vi "Scaling Test.vi"() -> ()   [LabVIEW 2016]
panel:
  out "Pre-Twos":bool[](array[boolean])
  out "Two's Complement":bool[](array[boolean])
  in  "Bit Count":u8=12
  out "Raw U64":u64 format="%064b"
  in  "Direction":bool
  in  "Raw":u16[](array[numeric]) format="%016b"
  in  "Scaled":dbl
  in  "Bit Offset":u8=2
  in  "LSB Resolution":dbl=1.0
  in  "2's Complement":bool
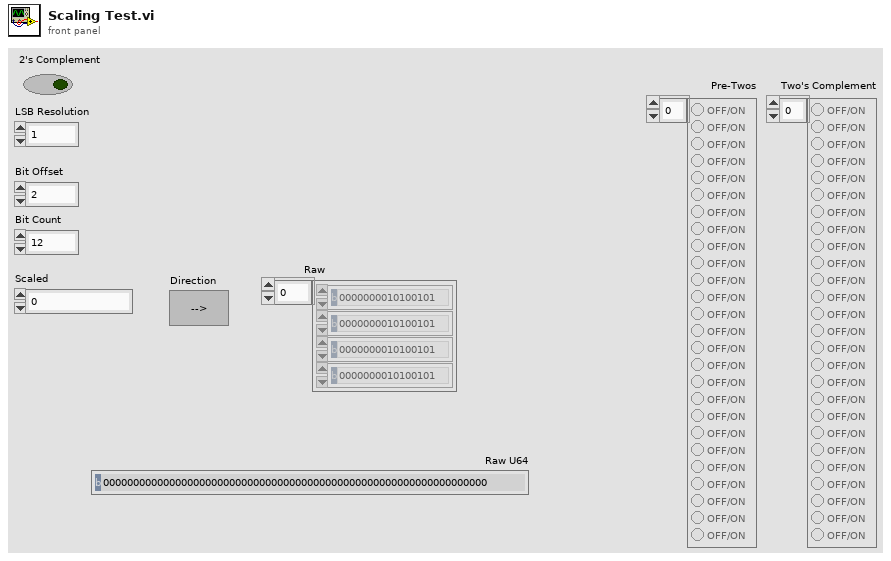
[diagram p1: front panel]
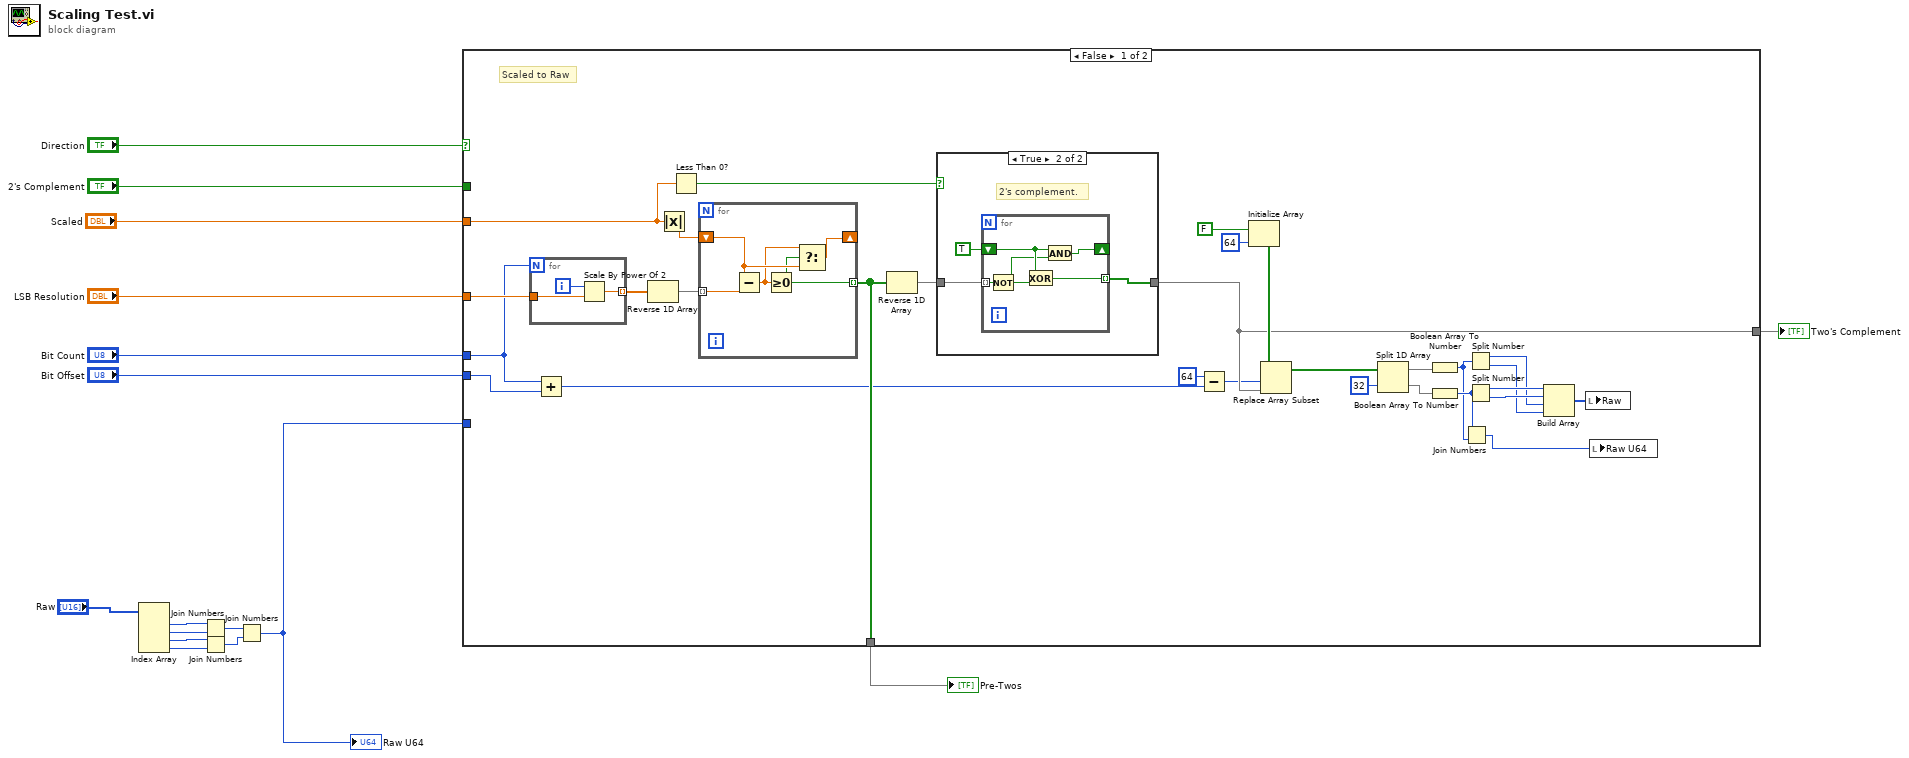
[diagram p0: block diagram]
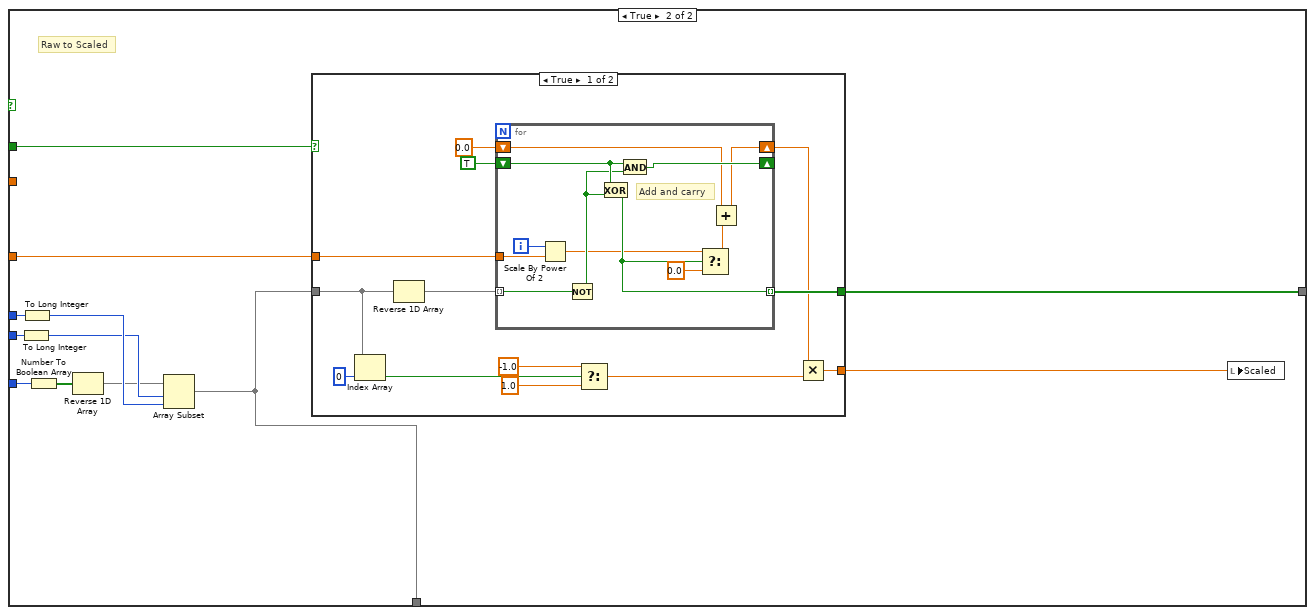
[diagram p3: hidden frame]
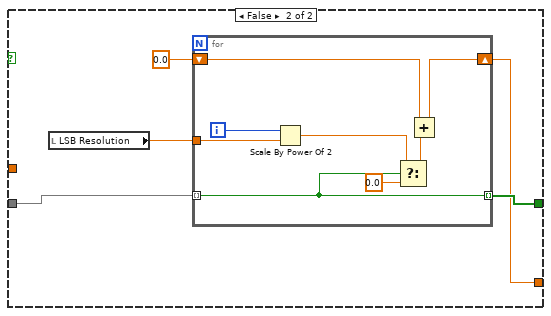
[diagram p4: hidden frame]
diagram:
  n1 = Index Array(array="Raw") -> (element #1=w6:u16, element #2=w7:u16, element #3=w4:u16, element #4=w5:u16)  [unwired: 4 in]
  n2 = Join Numbers(hi=w6, lo=w7) -> ((hi.lo)=w2:u32)
  n3 = Join Numbers(hi=w4, lo=w5) -> ((hi.lo)=w3:u32)
  n4 = Join Numbers(hi=w2, lo=w3) -> ((hi.lo)=w1:u64)
  "Raw U64" <- w1
  n5 = case shown="False" "Direction" {
    tunnel: "Bit Offset" -> [w27 w74]
    tunnel: w1 -> [_ w67]
    tunnel: "Bit Count" -> [w28 w73]
    tunnel: [w29 w71] -> w14
    tunnel: "2's Complement" -> [_ w70]
    tunnel: [w31 w66] -> w12
    tunnel: "LSB Resolution" -> [w45 w65]
    tunnel: "Scaled" -> [w42 _]
    frame False {
      # "Scaled to Raw"
      n6 = for {
        N: w28 -> [_]
        tunnel: w45 -> [w62]
        tunnel: [w60] -> w33 mode=indexing
        i -> [w61]
        n7 = Scale By Power Of 2(n=w61, x=w62) -> (x*2^n=w60:dbl)
      }
      n8 = Add(x=w28, y=w27) -> (x+y=w25:u8)
      n9 = Reverse 1D Array(array=w33) -> (reversed array=w32:dbl[])
      n10 = Absolute Value(x=w42) -> (abs(x)=w44:dbl)
      n11 = Less Than 0?(x=w42) -> (x < 0?=w43:bool)
      n12 = for {
        tunnel: w32 -> [w59] mode=indexing
        shift-right: [w57] -> _
        shift-left: w44 -> [w58]
        tunnel: [w56] -> w31 mode=indexing
        n13 = Subtract(x=w58, y=w59) -> (x-y=w55:dbl)
        n14 = Greater Or Equal To 0?(x=w55) -> (x >= 0?=w56:bool)
        n15 = Select(t=w55, s=w56, f=w58) -> (s? t:f=w57:dbl)
      }
      n16 = Reverse 1D Array(array=w31) -> (reversed array=w30:bool[])
      n17 = case shown="True" w43 {
        tunnel: [w46 w47] -> w29
        tunnel: w30 -> [w46 w49]
        frame False {
        }
        frame True {
          # "2's complement."
          n18 = for {
            tunnel: w49 -> [w54] mode=indexing
            shift-right: [w52] -> _
            shift-left: TRUE -> [w53]
            tunnel: [w51] -> w47 mode=indexing
            n19 = Not(x=w54) -> (.not. x?=w50:bool)
            n20 = Exclusive Or(1:w50, 2:w53) -> (0:w51:bool)
            n21 = And(x=w53, y=w50) -> (x .and. y?=w52:bool)
          }
        }
      }
      n22 = Subtract(x=u8 64 ("dimension size"), y=w25) -> (x-y=w24:u8)
      n23 = Initialize Array(FALSE, 64 ("dimension size")) -> (w39:bool[])
      n24 = Replace Array Subset(array=w39, new element=w29, index=w24) -> (w38:bool[])
      n25 = Split 1D Array(array=w38, index=32) -> (first subarray=w34:bool[], second subarray=w35:bool[])
      n26 = Boolean Array To Number(Boolean array=w34) -> (number=w18:u32)
      n27 = Boolean Array To Number(Boolean array=w35) -> (number=w19:u32)
      n28 = Join Numbers(hi=w19, lo=w18) -> ((hi.lo)=w17:u64)
      n29 = Split Number(x=w18) -> (hi(x)=w21:u16, lo(x)=w20:u16)
      n30 = Split Number(x=w19) -> (hi(x)=w23:u16, lo(x)=w22:u16)
      n31 = Build Array(w23, w22, w21, w20) -> (w36:u16[])
      n32 = local write "Raw"(w36) -> ()
      n33 = local write "Raw U64"(w17) -> ()
    }
    frame True {
      # "Raw to Scaled"
      n34 = To Long Integer(number=w74) -> (32bit integer=w69:i32)
      n35 = To Long Integer(number=w73) -> (32bit integer=w72:i32)
      n36 = Number To Boolean Array(number=w67) -> (Boolean array=w64:bool[])
      n37 = Reverse 1D Array(array=w64) -> (reversed array=w63:bool[])
      n38 = Array Subset(array=w63, index=w69, length=w72) -> (w66:bool[])
      n39 = case shown="True" w70 {
        tunnel: [w82 w104] -> w71
        tunnel: w66 -> [w77 w103]
        tunnel: [w83 w100] -> w68
        tunnel: w65 -> [w78 _]
        frame True {
          n40 = Index Array(array=w77, index=0) -> (element=w87:bool)
          n41 = Reverse 1D Array(array=w77) -> (reversed array=w75:bool[])
          n42 = for {
            tunnel: [w95] -> w82 mode=indexing
            tunnel: w75 -> [w99] mode=indexing
            shift-right: [w97] -> _
            shift-left: TRUE -> [w98]
            tunnel: w78 -> [w90]
            shift-right: [w93] -> w79
            shift-left: 0.0 -> [w92]
            i -> [w88]
            # "Add and carry"
            n43 = Scale By Power Of 2(n=w88, x=w90) -> (x*2^n=w89:dbl)
            n44 = Not(x=w99) -> (.not. x?=w96:bool)
            n45 = Exclusive Or(1:w96, 2:w98) -> (0:w95:bool)
            n46 = And(x=w98, y=w96) -> (x .and. y?=w97:bool)
            n47 = Select(t=w89, s=w95, f=0.0) -> (s? t:f=w91:dbl)
            n48 = Add(x=w92, y=w91) -> (x+y=w93:dbl)
          }
          n49 = Select(t=-1.0, s=w87, f=1.0) -> (s? t:f=w84:dbl)
          n50 = Multiply(x=w79, y=w84) -> (x*y=w83:dbl)
        }
        frame False {
          n51 = local read "LSB Resolution"() -> (w102:dbl)
          n52 = for {
            tunnel: [w109] -> w104 mode=indexing
            tunnel: w103 -> [w109] mode=indexing
            tunnel: w102 -> [w108]
            shift-right: [w105] -> w100
            shift-left: 0.0 -> [w111]
            i -> [w106]
            n53 = Scale By Power Of 2(n=w106, x=w108) -> (x*2^n=w107:dbl)
            n54 = Select(t=w107, s=w109, f=0.0) -> (s? t:f=w110:dbl)
            n55 = Add(x=w111, y=w110) -> (x+y=w105:dbl)
          }
        }
      }
      n56 = local write "Scaled"(w68) -> ()
    }
  }
  "Two's Complement" <- w14
  "Pre-Twos" <- w12
